vi "随机二维数组.vi"() -> (0 "数组":i16[][](array[numeric]))   [LabVIEW 2017]
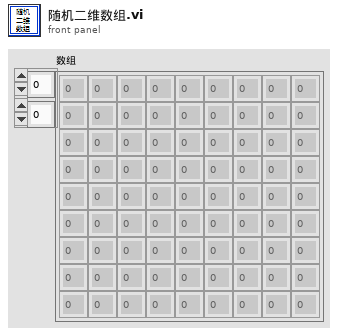
[diagram p1: front panel]
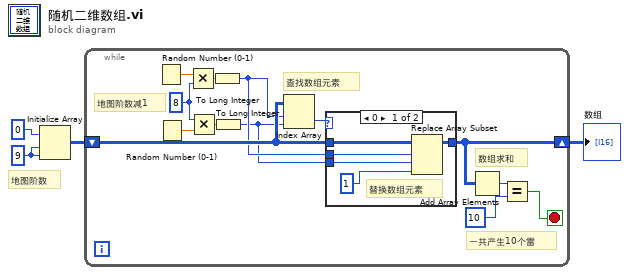
[diagram p0: block diagram]
diagram:
  w1 = 9
  # "地图阶数"
  n1 = Initialize Array(0, w1, w1) -> (w3:i32[][])
  n2 = while {
    shift-right: [w7] -> w4
    shift-left: w3 -> [w12]
    stop <- w6 stop-if-true
    w13 = 8
    # "数组求和"
    # "查找数组元素"
    # "一共产生10个雷"
    # "地图阶数减1"
    n3 = Random Number (0-1)() -> (number: 0 to 1=w14:dbl)
    n4 = Random Number (0-1)() -> (number: 0 to 1=w17:dbl)
    n5 = Multiply(x=w14, y=w13) -> (x*y=w15:dbl)
    n6 = Multiply(x=w13, y=w17) -> (x*y=w16:dbl)
    n7 = To Long Integer(number=w15) -> (32bit integer=w11:i32)
    n8 = To Long Integer(number=w16) -> (32bit integer=w10:i32)
    n9 = Index Array(array=w12, index (row)=w11, index (col)=w10) -> (element=w5:i32)
    n10 = case shown="0" w5 {
      tunnel: [w22 w23] -> w7
      tunnel: w12 -> [w21 w23]
      tunnel: w11 -> [w20 _]
      tunnel: w10 -> [w19 _]
      frame 0 {
        # "替换数组元素"
        n11 = Replace Array Subset(array=w21, new element=1, index (row)=w20, index (col)=w19) -> (w22:i32[][])
      }
      frame 1, Default {
      }
    }
    n12 = Add Array Elements(numeric array=w7) -> (sum=w9:i32)
    n13 = Equal?(x=w9, y=10) -> (x = y?=w6:bool)
  }
  "数组" <- w4
